vi "exmpl_Append_to_Log.vi"(8 "error in (no error)":errorcluster, 10 "Log Array in":string[](array[string]), 11 "Log Message":string) -> (0 "error out":errorcluster, 2 "Log Array out":string[](array[string]))   [LabVIEW 2013, in "daqio minimal.lvlib"]
uses:
  daqio minimal.lvlib
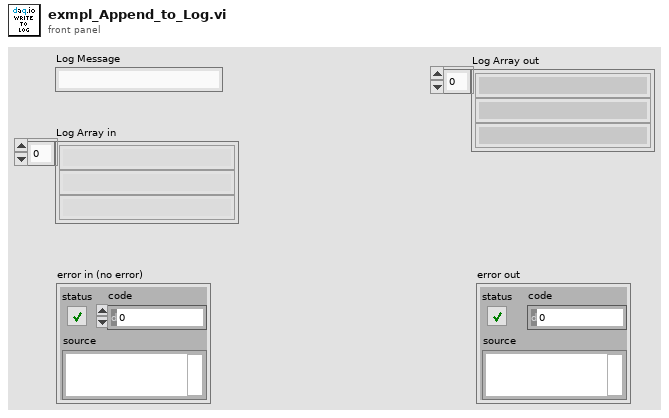
[diagram p1: front panel]
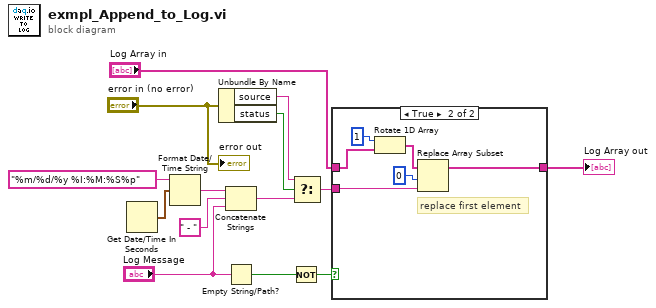
[diagram p0: block diagram]
diagram:
  n1 = Get Date/Time In Seconds() -> (seconds since 1Jan1904=w7:timestamp)
  n2 = Format Date/Time String(time format string (%c)="%m/%d/%y %I:%M:%S%p", seconds (now)=w7) -> (date/time string=w9:string)  [unwired: 1 in]
  n3 = Unbundle By Name("error in (no error)") -> ("source"=w3:string, "status"=w4:bool)
  n4 = Concatenate Strings(w9, " - " ("string"), "Log Message") -> (w8:string)
  n5 = Empty String/Path?(string/path="Log Message") -> (empty?=w14:bool)
  n6 = Not(x=w14) -> (.not. x?=w13:bool)
  n7 = Select(t=w3, s=w4, f=w8) -> (s? t:f=w5:string)
  n8 = case shown="True" w13 {
    tunnel: w5 -> [_ w21]
    tunnel: "Log Array in" -> [w15 w16]
    tunnel: [w15 w17] -> w1
    frame False {
    }
    frame True {
      # "replace first element"
      n9 = Rotate 1D Array(1:w16, 2:1 ("n")) -> (0:w18:string[])
      n10 = Replace Array Subset(array=w18, new element=w21, index=0) -> (w17:string[])
    }
  }
  "Log Array out" <- w1
  "error out" <- "error in (no error)"
